vi "XML Reader Close.vi"(8 "error in":errorcluster, 11 "XML Reader In":T1) -> (0 "error out":errorcluster)   [LabVIEW 2017, in "Pathloss XML Reader.lvlib"]
uses:
  Pathloss XML Reader.lvlib
  Controls/XML Reader Data Ref.ctl
  Controls/XML Reader Data.ctl
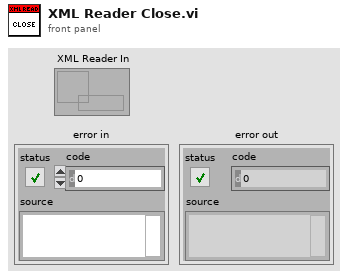
[diagram p1: front panel]
types:
  T1 = typedef "Pathloss XML Reader.lvlib/XML Reader Data Ref.ctl" = refnum<data-value>
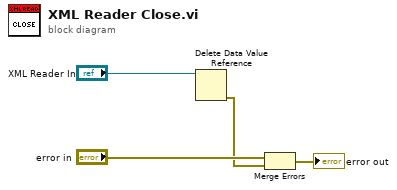
[diagram p0: block diagram]
diagram:
  n1 = Delete Data Value Reference(data value reference="XML Reader In") -> (error out=w1:errorcluster)  [unwired: 1 in, 1 out]
  n2 = Merge Errors("error in", w1) -> (→"error out":errorcluster)
